vi "Camera Serial Number Map.vi"(7 "Update":bool, 9 "Serial Number":u32, 11 "map":map{u32, T1}(c390)) -> (3 "Camera Name":T1)   [LabVIEW 2025]
uses:
  <vilib>/userDefined/High Color/IMAQdx.ctl
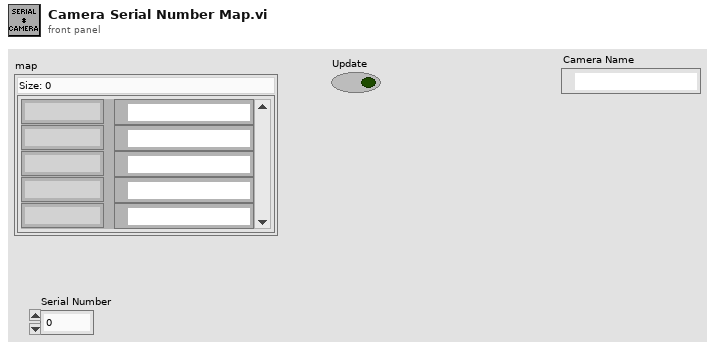
[diagram p1: front panel]
types:
  T1 = typedef "IMAQdx.ctl" = refnum<k21>
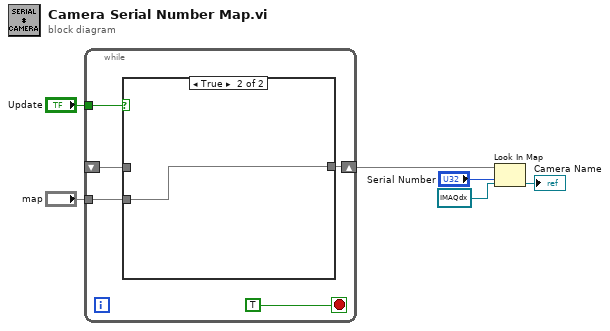
[diagram p0: block diagram]
diagram:
  n1 = while {
    tunnel: "Update" -> [w10]
    tunnel: "map" -> [w9]
    shift-right: [w8] -> w5
    shift-left: _ -> [w7]
    stop <- TRUE stop-if-true
    n2 = case shown="True" w10 {
      tunnel: w9 -> [_ w13]
      tunnel: [w12 w13] -> w8
      tunnel: w7 -> [w12 _]
      frame False {
      }
      frame True {
      }
    }
  }
  n3 = Look In Map(map=w5, key="Serial Number", default value=T1 refnum) -> (value=→"Camera Name":T1)  [unwired: 1 out]
